vi "Vector Elementwise Multiplication_v1.1.vi"(1 "Matrix 1":T1, 2 "Matrix in":T1) -> (0 "elementwise product":T1)   [LabVIEW 2020]
uses:
  <vilib>/Analysis/Matrix/Datatypes/RealMatrix.ctl
  <vilib>/Analysis/Matrix/Numeric/Conversions/Matrix To Array - RM.vi
  <vilib>/Analysis/Matrix/Numeric/Conversions/Array To Matrix - RA2.vi
  <vilib>/Analysis/Matrix/NI_Matrix.lvlib
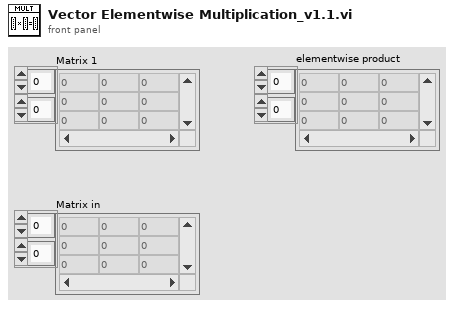
[diagram p1: front panel]
types:
  T1 = typedef "NI_Matrix.lvlib/RealMatrix.ctl" = dbl[][]
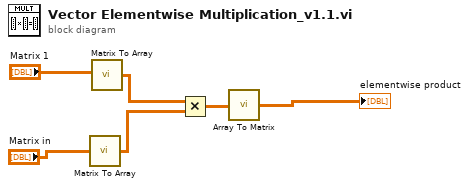
[diagram p0: block diagram]
diagram:
  n1 = call-poly <vilib>:"Matrix To Array.vi"("Real Matrix"="Matrix in") -> ("Real 2D Array"=w5:dbl[][])
  n2 = call-poly <vilib>:"Matrix To Array.vi"("Real Matrix"="Matrix 1") -> ("Real 2D Array"=w4:dbl[][])
  n3 = Multiply(x=w4, y=w5) -> (x*y=w6:dbl[][])
  n4 = call-poly <vilib>:"Array To Matrix.vi"("Real 2D Array"=w6) -> ("Real Matrix"=→"elementwise product":T1)
